vi "wait for hold mercury.vi"(8 "error in (no error)":errorcluster, 10 "Device on PSU":string, 11 "VISA resource name":refnum<visa-resource-name>) -> (0 "error out":errorcluster, 3 "VISA resource name 2":refnum<visa-resource-name>)   [LabVIEW 2018]
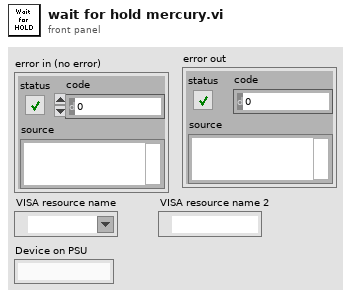
[diagram p1: front panel]
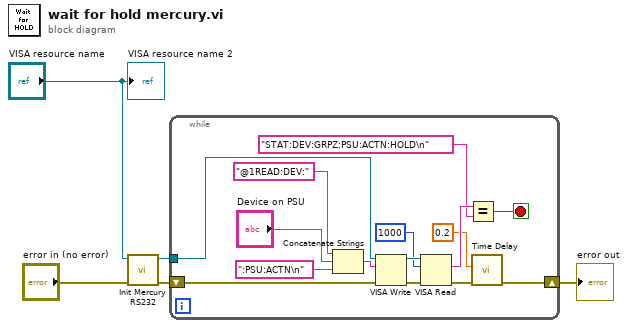
[diagram p0: block diagram]
diagram:
  n1 = call "Init Mercury RS232.vi"("error in (no error)"="error in (no error)", "VISA resource name"="VISA resource name") -> ("error out"=w4:errorcluster, "VISA resource name out"=w2:refnum<visa-resource-name>)  [unwired: 8 in]
  n2 = while {
    shift-right: [w7] -> w1
    shift-left: w4 -> [w20]
    tunnel: w2 -> [w19]
    stop <- w8 stop-if-true
    n3 = Concatenate Strings("@1READ:DEV:" ("write buffer"), "Device on PSU", ":PSU:ACTN\n" ("string")) -> (w15:string)
    n4 = VISA Write(VISA resource name=w19, write buffer=w15, error in (no error)=w20) -> (VISA resource name out=w12:refnum<visa-resource-name>, error out=w14:errorcluster)  [unwired: 1 out]
    n5 = VISA Read(VISA resource name=w12, byte count=u32 1000, error in (no error)=w14) -> (read buffer=w10:string, error out=w13:errorcluster)  [unwired: 2 out]
    n6 = Equal?(x=w10, y="STAT:DEV:GRPZ:PSU:ACTN:HOLD\n") -> (x = y?=w8:bool)
    n7 = call "Time Delay"("error in (no error)"=w13, "Delay Time (s)"=0.2) -> ("error out"=w7:errorcluster)  [unwired: 9 in]
  }
  "error out" <- w1
  "VISA resource name 2" <- "VISA resource name"
